vi "Init.vi"(8 "error in (no error)":errorcluster) -> (0 "error out":errorcluster, 3 "Controller out":refnum<class "Controller.lvclass">)   [LabVIEW 2020, in "Controller.lvclass"]
uses:
  Controller.lvclass
  controls/Module response.ctl
  Controller.lvclass/Controller.ctl
  Logging/Logging.lvclass
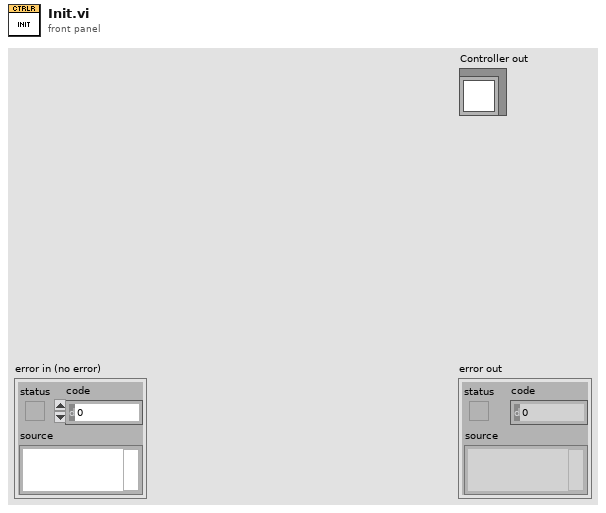
[diagram p1: front panel]
types:
  T1 = typedef "Module response.ctl" = cluster{"ID":string, "Response":variant}
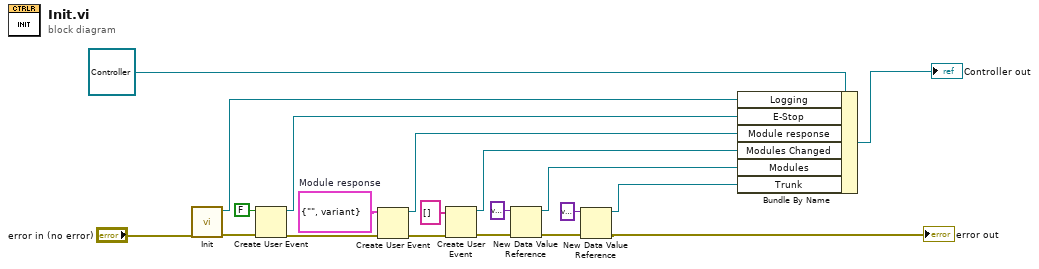
[diagram p0: block diagram]
diagram:
  w3 = T1 {"ID"="", "Response"=variant}  # Module response
  n1 = call "Init.vi"("error in (no error)"="error in (no error)") -> ("error out"=w7:errorcluster, "Logging out"=w17:refnum<class "Logging.lvclass">)  [unwired: 9 in]
  n2 = Create User Event(user event datatype=FALSE ("Stop Event"), error in=w7) -> (user event=w6:refnum<user-event>, error out=w4:errorcluster)
  n3 = Create User Event(user event datatype=w3, error in=w4) -> (user event=w2:refnum<user-event>, error out=w5:errorcluster)
  n4 = Create User Event(user event datatype=string[] [] ("Names"), error in=w5) -> (user event=w11:refnum<user-event>, error out=w13:errorcluster)
  n5 = New Data Value Reference(data value=variant, error in=w13) -> (data value reference=w10:refnum<data-value>, error out=w14:errorcluster)
  n6 = New Data Value Reference(data value=variant, error in=w14) -> (data value reference=w9:refnum<data-value>, error out=→"error out":errorcluster)
  n7 = Bundle By Name(cluster=refnum<class "Controller.lvclass"> refnum ("Controller in"), "Logging"=w17, "E-Stop"=w6, "Module response"=w2, "Modules Changed"=w11, "Modules"=w10, "Trunk"=w9) -> (→"Controller out":refnum<class "Controller.lvclass">)
